vi "Draw Mean Style.vi"(8 "error in (no error)":errorcluster, 11 "Graph Manager in":refnum<class "Graph Manager.lvclass">) -> (0 "error out":errorcluster, 3 "Graph Manager out":refnum<class "Graph Manager.lvclass">)   [LabVIEW 2016, in "Graph Manager.lvclass"]
uses:
  Graph Manager.lvclass
  Graph Manager.lvclass/Graph Manager.ctl
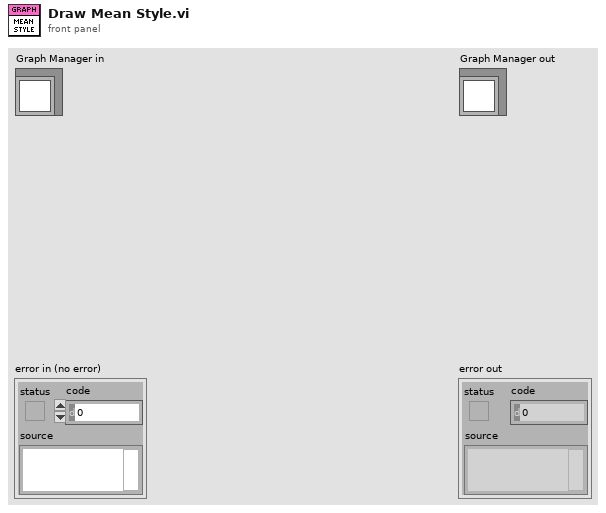
[diagram p1: front panel]
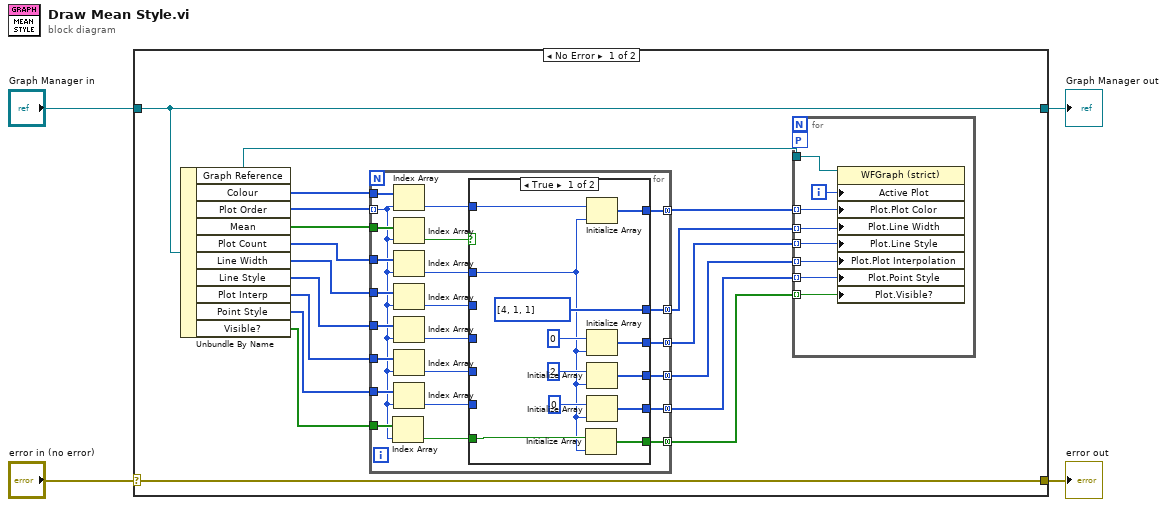
[diagram p0: block diagram]
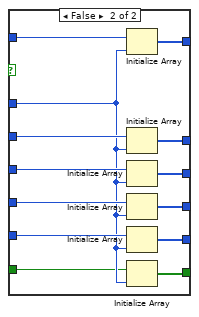
[diagram p2: hidden frame]
diagram:
  n1 = case shown="No Error" "error in (no error)" {
    selector: "error in (no error)" -> [w22 w80]
    tunnel: [w22 w80] -> w3
    tunnel: [w21 w79] -> w1
    tunnel: "Graph Manager in" -> [w21 w79]
    frame No Error {
      n2 = Unbundle By Name(w21) -> ("Graph Reference"=w20:refnum<vi>, "Colour"=w19:u32[], "Plot Order"=w17:i32[], "Mean"=w15:bool[], "Plot Count"=w14:i32[], "Line Width"=w13:u8[], "Line Style"=w12:u8[], "Plot Interp"=w11:u8[], "Point Style"=w10:u8[], "Visible?"=w6:bool[])
      n3 = for {
        tunnel: w19 -> [w44]
        tunnel: [w45] -> w18 mode=concatenating
        tunnel: w17 -> [w25] mode=indexing
        tunnel: [w42] -> w16 mode=concatenating
        tunnel: w15 -> [w41]
        tunnel: w14 -> [w40]
        tunnel: w13 -> [w39]
        tunnel: w12 -> [w38]
        tunnel: w11 -> [w37]
        tunnel: w10 -> [w36]
        tunnel: [w29] -> w9 mode=concatenating
        tunnel: [w28] -> w8 mode=concatenating
        tunnel: [w27] -> w7 mode=concatenating
        tunnel: w6 -> [w26]
        tunnel: [w23] -> w5 mode=concatenating
        n4 = Index Array(array=w26, index=w25) -> (element=w24:bool)
        n5 = Index Array(array=w44, index=w25) -> (element=w43:u32)
        n6 = Index Array(array=w41, index=w25) -> (element=w35:bool)
        n7 = Index Array(array=w40, index=w25) -> (element=w30:i32)
        n8 = Index Array(array=w39, index=w25) -> (element=w34:u8)
        n9 = Index Array(array=w38, index=w25) -> (element=w33:u8)
        n10 = Index Array(array=w37, index=w25) -> (element=w32:u8)
        n11 = Index Array(array=w36, index=w25) -> (element=w31:u8)
        n12 = case shown="True" w35 {
          tunnel: [w57 w70] -> w45
          tunnel: w43 -> [w56 w69]
          tunnel: [u8[] [4, 1, 1] ("Line Width") w64] -> w42
          tunnel: w34 -> [_ w68]
          tunnel: w33 -> [_ w67]
          tunnel: w32 -> [_ w66]
          tunnel: w31 -> [_ w65]
          tunnel: w30 -> [w47 w60]
          tunnel: [w49 w63] -> w29
          tunnel: [w50 w62] -> w28
          tunnel: [w51 w61] -> w27
          tunnel: w24 -> [w48 w59]
          tunnel: [w46 w58] -> w23
          frame True {
            n13 = Initialize Array(w48, w47) -> (w46:bool[])
            n14 = Initialize Array(w56, w47) -> (w57:u32[])
            n15 = Initialize Array(u8 0 ("element"), w47) -> (w49:u8[])
            n16 = Initialize Array(u8 2 ("element"), w47) -> (w50:u8[])
            n17 = Initialize Array(u8 0 ("element"), w47) -> (w51:u8[])
          }
          frame False {
            n18 = Initialize Array(w69, w60) -> (w70:u32[])
            n19 = Initialize Array(w68, w60) -> (w64:u8[])
            n20 = Initialize Array(w67, w60) -> (w63:u8[])
            n21 = Initialize Array(w66, w60) -> (w62:u8[])
            n22 = Initialize Array(w65, w60) -> (w61:u8[])
            n23 = Initialize Array(w59, w60) -> (w58:bool[])
          }
        }
      }
      n24 = for {
        tunnel: w20 -> [w78]
        workers-P: _ -> [_]
        tunnel: w18 -> [w76] mode=indexing
        tunnel: w16 -> [w75] mode=indexing
        tunnel: w9 -> [w74] mode=indexing
        tunnel: w8 -> [w73] mode=indexing
        tunnel: w7 -> [w72] mode=indexing
        tunnel: w5 -> [w71] mode=indexing
        i -> [w77]
        n25 = property class="WFGraph (strict)"(reference=w78, "Active Plot"=w77, "Plot.Plot Color"=w76, "Plot.Line Width"=w75, "Plot.Line Style"=w74, "Plot.Plot Interpolation"=w73, "Plot.Point Style"=w72, "Plot.Visible?"=w71) -> ()  [unwired: 1 in, 2 out]
      }
    }
    frame Error {
    }
  }
  "error out" <- w3
  "Graph Manager out" <- w1
